vi "Read Modules Timing Source.vi"(8 "error in":errorcluster, 11 "Engine Parent in":refnum<class "Engine Parent Editor Node.lvclass">) -> (0 "error out":errorcluster, 2 "timing masters":string[](array[string]), 3 "Engine Parent out":refnum<class "Engine Parent Editor Node.lvclass">)   [LabVIEW 2013, in "PL Framework Configuration Tool.lvlib" / "Engine Parent Editor Node.lvclass"]
uses:
  Engine Parent Editor Node.lvclass
  <vilib>/NI/Configuration Framework/Node/NISE_CEF_Node.lvclass/NISE_CEF_Node.ctl
  Module editor node/module editor node.lvclass
  <vilib>/NI/Tag Bus Module Framework/module configuration/timing source.ctl
  <vilib>/NI/Tag Bus Module Framework/module configuration/TBM module configuration.lvclass
  <vilib>/NI/Configuration Framework/Node/NISE_CEF_Node.lvclass
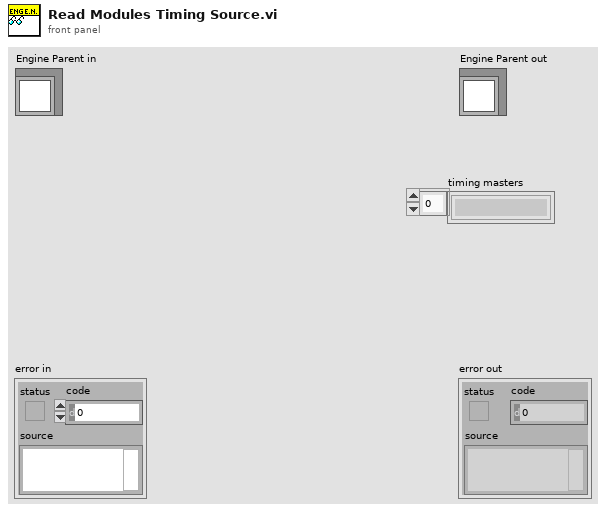
[diagram p1: front panel]
types:
  T1 = typedef "TBM module configuration.lvclass/timing source.ctl" = enum16{"None", "Custom Timing Source", "1 kHz Clock", "1 MHz Clock", "Synchronize to Scan Engine"}
  T2 = typedef "NISE_CEF_Node.lvclass/NodeRef.ctl" = refnum<data-value>
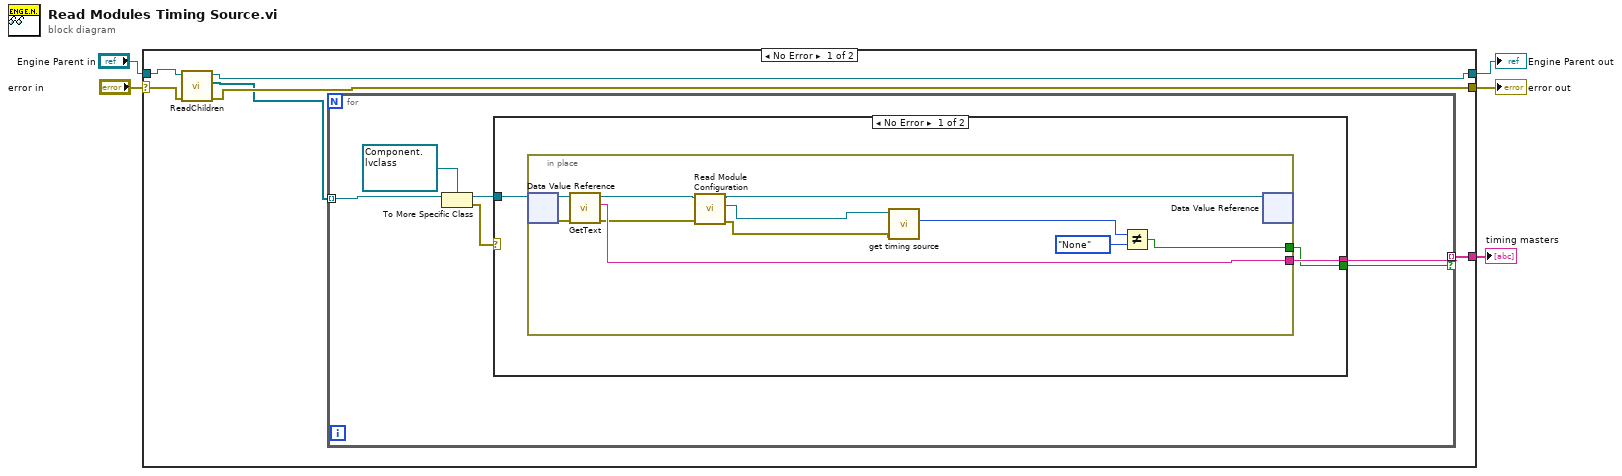
[diagram p0: block diagram]
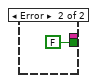
[diagram p2: hidden frame]
diagram:
  n1 = case shown="No Error" "error in" {
    selector: "error in" -> [w7 w33]
    tunnel: [w8 w33] -> w4
    tunnel: [w9 w34] -> w2
    tunnel: "Engine Parent in" -> [w10 w34]
    tunnel: [w11 _] -> w1
    frame No Error {
      n2 = call <vilib>:"ReadChildren.vi"("error in"=w7, "node in"=w10) -> ("error out"=w8:errorcluster, "output array"=w6:T2[], "node out"=w9:refnum<class "Engine Parent Editor Node.lvclass">)  [unwired: 7 in]
      n3 = for {
        tunnel: [w17] -> w11 mode=indexing if=w16
        tunnel: w6 -> [w13] mode=indexing
        n4 = To More Specific Class(target class=refnum<data-value> refnum ("data value reference"), reference=w13) -> (specific class reference=w15:refnum<data-value>, error out=w14:errorcluster)  [unwired: 1 in]
        n5 = case shown="No Error" w14 {
          tunnel: [w20 _] -> w17
          tunnel: [w19 FALSE] -> w16
          tunnel: w15 -> [w18 _]
          frame No Error {
            n6 = in-place {
              in-place-border: [w30] -> w19
              in-place-border: [w29] -> w20
              n7 = in-place-dvr #1(w18) -> (w31:refnum<class "module editor node.lvclass">, w22:errorcluster)
              n8 = call-dynamic "GetText.vi"("error in"=w22, "Module Editor Node in"=w31) -> ("error out"=w21:errorcluster, "text"=w29:string, "Module Editor Node out"=w28:refnum<class "module editor node.lvclass">)  [unwired: 5 in, 2 out]
              n9 = call "Read Module Configuration.vi"("error in"=w21, "Module Editor Node in"=w28) -> ("error out"=w24:errorcluster, "module configuration"=w25:refnum<class "TBM module configuration.lvclass">, "Module Editor Node out"=w27:refnum<class "module editor node.lvclass">)  [unwired: 7 in]
              n10 = call-dynamic "get timing source.vi"("error in"=w24, "module configuration in"=w25) -> ("timing source enum"=w23:T1)  [unwired: 7 in, 2 out]
              n11 = Not Equal?(x=w23, y=timing_source."None") -> (x != y?=w30:bool)
              n12 = in-place-dvr #1(w27) -> ()  [unwired: 2 out]
            }
          }
          frame Error {
          }
        }
      }
    }
    frame Error {
    }
  }
  "error out" <- w4
  "Engine Parent out" <- w2
  "timing masters" <- w1
